vi "Teleop_Alternate.vi"(10 "Match Info":T1={"Autonomous Elapsed Seconds"=0.0, "TeleOp Elapsed Seconds"=0.0, "Disabled Elapsed Seconds"=0.0, "Visited Autonomous"=FALSE, "Visited TeleOp"=FALSE, "Visited Disabled"=FALSE, "Autonomous Settings"={"Autonomous Style"=enum."Independent", "VI Refnum"=refnum}}, 11 "Call Context":T2=enum."Stop") -> ()   [LabVIEW 2015]
doc: "This VI is called for each TeleOp packet received from the DS where the robot is not disabled. It is often used to read from the joysticks and update I/O or to update setpoints for timed control loops. It should complete and return within 20 milliseconds or it may miss DS packets."
uses:
  <vilib>/Rock Robotics/WPI/DriverStation/WPI_DriverStationDerivedRobotMode.ctl
  <vilib>/Rock Robotics/WPI/DriverStation/WPI_DriverStationMatch Info.ctl
  <vilib>/Rock Robotics/WPI/Solenoid/WPI_SolenoidValue.ctl
  Typedef/XBox Buttons.ctl
  Typedef/XBox Axis.ctl
  <vilib>/Rock Robotics/WPI/Utilities/WPI_GetSetVariantRefNum.vi
  <vilib>/Rock Robotics/Network Tables/NT Write Boolean Array.vi
  <vilib>/Rock Robotics/Network Tables/NT Write Numeric Array.vi
  Robot Global Data.vi
  <vilib>/Rock Robotics/WPI/RobotDrive/WPI_RobotDriveArcadeDrive_Standard(NoSaturation).vi
  <vilib>/Rock Robotics/Network Tables/NT Write Number.vi
  <vilib>/Rock Robotics/Network Tables/NT Write String.vi
  <vilib>/Rock Robotics/WPI/Solenoid/WPI_SolenoidSetEnum.vi
  ArmController/ArmController.lvlib
panel:
  in  "Reset":bool
  out "Shifts":i32
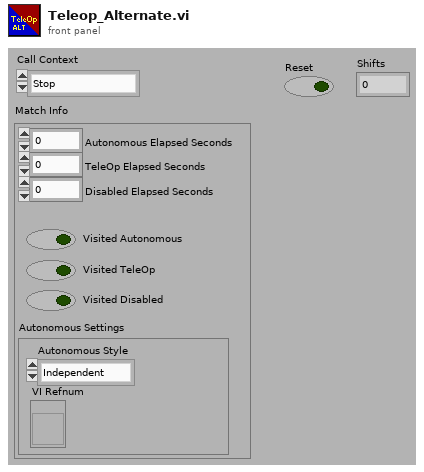
[diagram p1: front panel]
types:
  T1 = typedef "WPI_DriverStationMatch Info.ctl" = cluster{"Autonomous Elapsed Seconds":dbl, "TeleOp Elapsed Seconds":dbl, "Disabled Elapsed Seconds":dbl, "Visited Autonomous":bool, "Visited TeleOp":bool, "Visited Disabled":bool, "Autonomous Settings":cluster{"Autonomous Style":enum16{"Iterative", "Independent"}, "VI Refnum":refnum<vi>}}
  T2 = typedef "WPI_DriverStationDerivedRobotMode.ctl" = enum16{"Init", "Execute", "Stop"}
  T3 = typedef "WPI_SolenoidValue.ctl" = enum16{"Off", "On", "Forward", "Reverse"}
  T4 = typedef "WPI_JoystickDevRef.ctl" = cluster{"Device":T5}
  T5 = typedef "WPI_JoystickDeviceEnum.ctl" = enum16{"USB 0", "USB 1", "USB 2", "USB 3", "USB 4", "USB 5"}
  T6 = typedef "WPI_RobotDriveDevRef.ctl" = cluster{"DevStatus":errorcluster, "Motors[]":T7[], "Square Inputs":bool, "Max Output":dbl}
  T7 = typedef "WPI_MotorControlDeviceRef.ctl" = cluster{"DeviceStatus":errorcluster, "Type":T8, "PWM":cluster{"PWM Channel":T9, "DeadBand":T10}, "CAN":cluster{"Device Number":u8, "Control Mode":T11, "Semaphore":T12, "Max Vout":dbl, "TalonSRX Control Mode":T13}, "Invert":bool}
  T8 = typedef "WPI_MotorControlType.ctl" = enum16{"PWM", "CAN", "CANTalonSRX"}
  T9 = typedef "FPGA_DIOPWMChannel.ctl" = enum8{"PWM 0", "PWM 1", "PWM 2", "PWM 3", "PWM 4", "PWM 5", "PWM 6", "PWM 7", "PWM 8", "PWM 9", "PWM MXP 0", "PWM MXP 1", "PWM MXP 2", "PWM MXP 3", "PWM MXP 4", "PWM MXP 5", "PWM MXP 6", "PWM MXP 7", "PWM MXP 8", "PWM MXP 9", "Invalid"}
  T10 = typedef "WPI_PWMDeadband.ctl" = cluster{"Name":string, "maxPositivePwm":i32, "minPositivePwm":i32, "centerPwm":i32, "maxNegativePwm":i32, "minNegativePwm":i32, "angularRange":u16}
  T11 = typedef "WPI_CANJaguar_ControlMode.ctl" = enum8{"Percent VBus", "Current", "Speed", "Position", "Voltage"}
  T12 = typedef "Semaphore RefNum" = refnum<k1>
  T13 = typedef "WPI_CANTalonSRX_APIControlMode.ctl" = enum8{"Percent VBus", "Speed", "Position", "Slave", "Unchanged / Invalid", "Voltage Compensation", "Current", "Motion Profile"}
  T14 = typedef "XBox Axis.ctl" = enum16{"Left X", "Left Y", "Left Trigger", "Right Trigger", "Right X", "Right Y"}
  T15 = typedef "XBox Buttons.ctl" = enum16{"A", "B", "X", "Y", "Left Bumper", "Right Bumper", "Back", "Start", "Left Joystick", "Right Joystick"}
  T16 = typedef "ArmController.lvlib/ArmRef.ctl" = cluster{"Pot":T17, "ArmMotor":T7, "Queue":refnum<queue>, "Setpoint":dbl, "Manual":bool, "output range":cluster{"output high":dbl, "output low":dbl}, "PID gains":cluster{"proportional gain (Kc)":dbl, "integral time (Ti, min)":dbl, "derivative time (Td, min)":dbl}}
  T17 = typedef "WPI_PotentiometerDevRef.ctl" = cluster{"DevStatus":errorcluster, "Analog Channel":T18, "Invert Output":bool}
  T18 = typedef "FPGA_AIChannel.ctl" = enum8{"AI 0", "AI 1", "AI 2", "AI 3", "AI MXP 0", "AI MXP 1", "AI MXP 2", "AI MXP 3", "Invalid"}
  T19 = cluster{"Down":dbl, "Pickup":dbl, "Shoot":dbl, "Turtle":dbl, "Intake Transfer":dbl}
  T20 = typedef "WPI_SolenoidDevRef.ctl" = cluster{"DevStatus":errorcluster, "Pneumatics Control Module":u8, "Forward Solenoid Channel":T21, "Reverse Solenoid Channel":T21}
  T21 = typedef "WPI_SolenoidChannel.ctl" = enum8{"Solenoid 0", "Solenoid 1", "Solenoid 2", "Solenoid 3", "Solenoid 4", "Solenoid 5", "Solenoid 6", "Solenoid 7", "Invalid"}
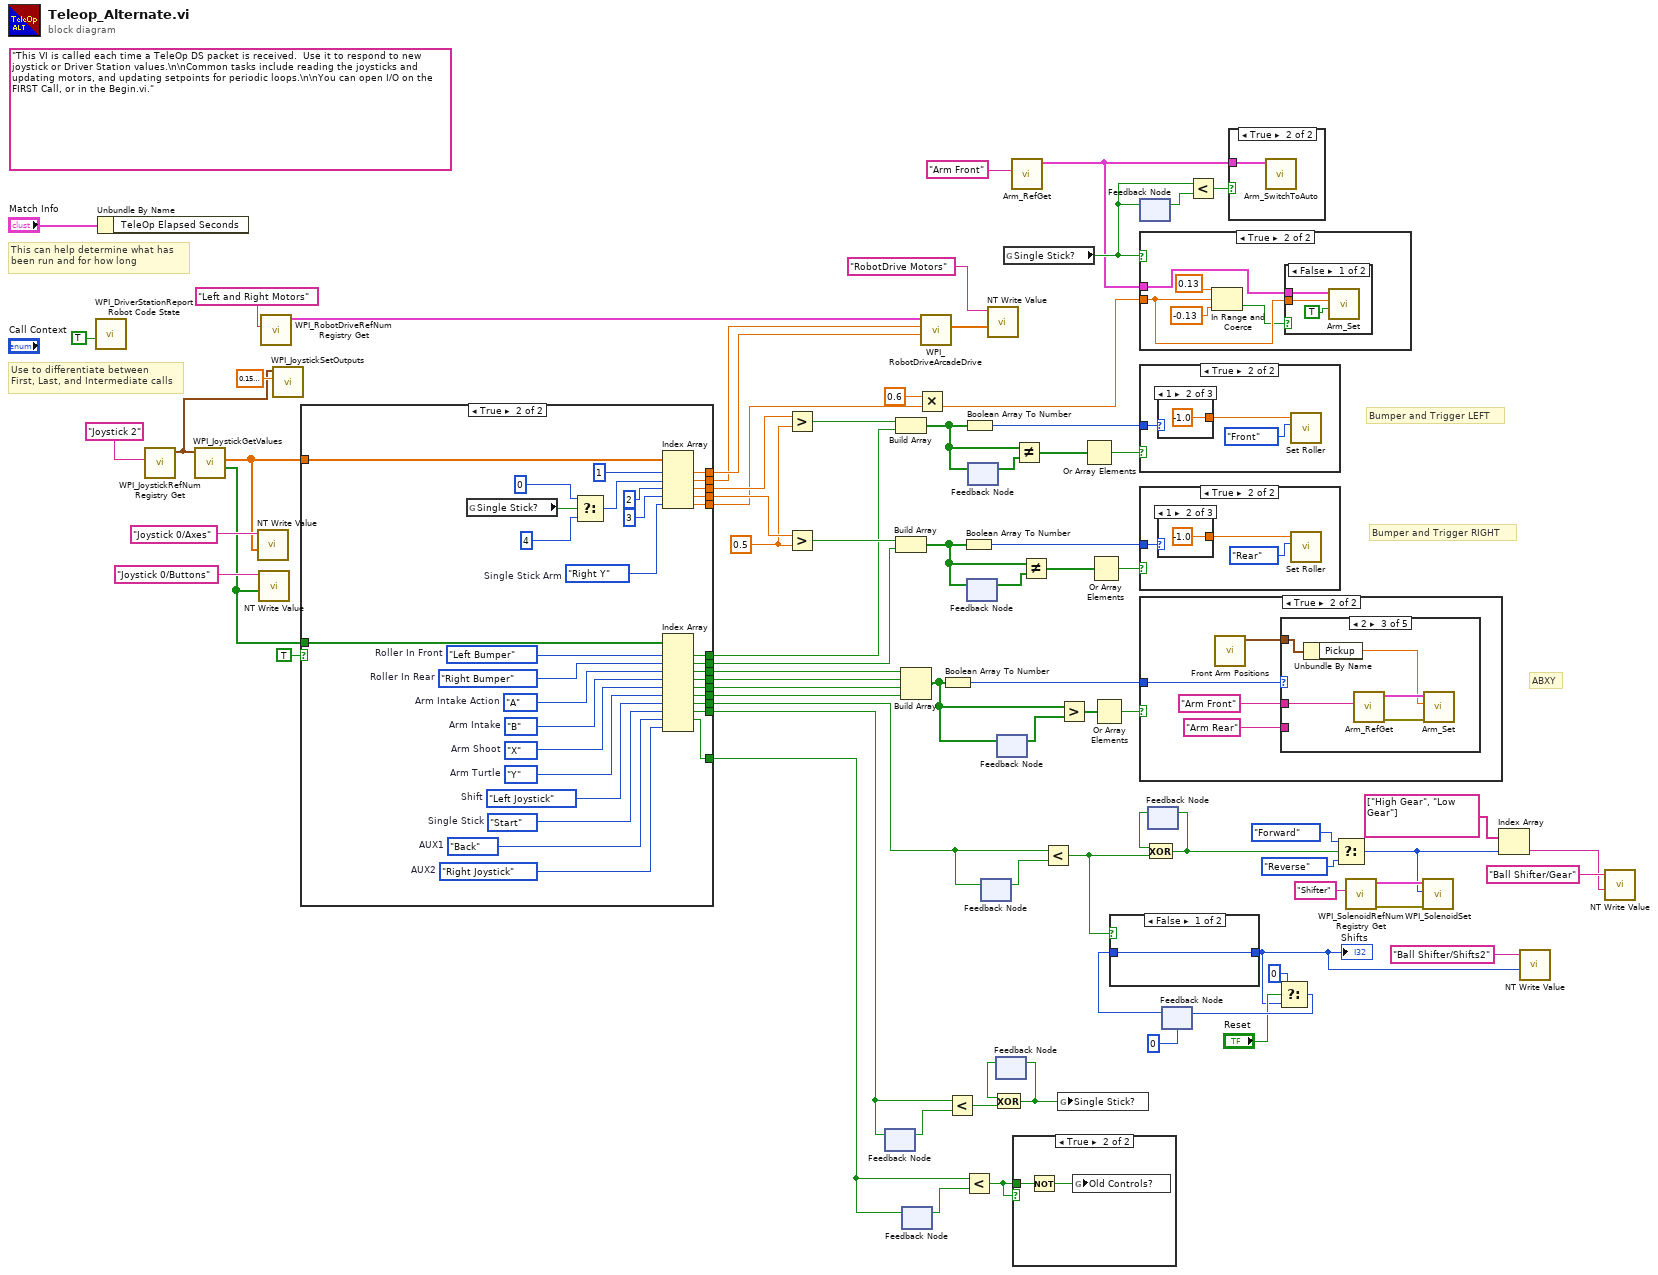
[diagram p0: block diagram]
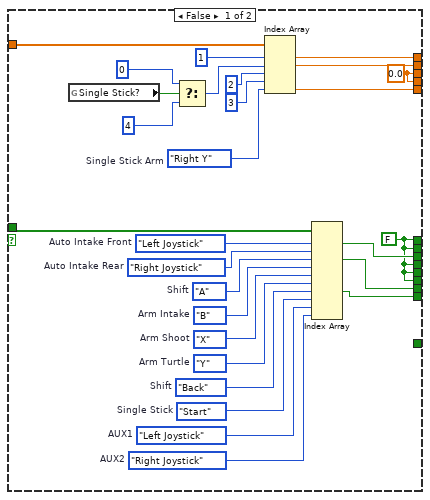
[diagram p3: hidden frame]
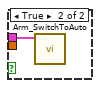
[diagram p6: hidden frame]
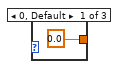
[diagram p8: hidden frame]
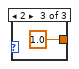
[diagram p9: hidden frame]
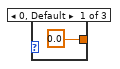
[diagram p11: hidden frame]
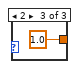
[diagram p12: hidden frame]
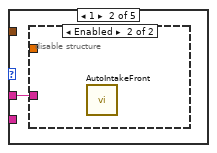
[diagram p15: hidden frame]
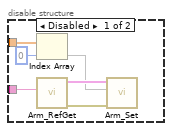
[diagram p16: hidden frame]
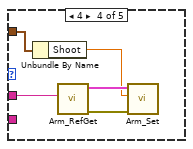
[diagram p17: hidden frame]
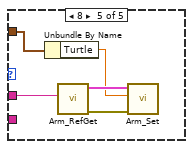
[diagram p18: hidden frame]
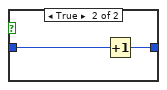
[diagram p19: hidden frame]
diagram:
  w44 = 0.5 ("x")
  (unwired) "This VI is called each time a TeleOp DS packet is received.  Use it to respond to new joystick or Driver Station values.\n\nCommon tasks include reading the joysticks and updating motors, and updating setpoints for periodic loops.\n\nYou can open I/O on the FIRST Call, or in the Begin.vi."
  # "ABXY"
  # "Bumper and Trigger RIGHT"
  # "Bumper and Trigger LEFT"
  # "Use to differentiate between\nFirst, Last, and Intermediate calls"
  # "This can help determine what has\nbeen run and for how long"
  n1 = call <vilib>:"WPI_DriverStationReport Robot Code State.vi"("TeleOp"=TRUE ("Autonomous")) -> ()  [unwired: 10 in, 1 out]
  n2 = Unbundle By Name("Match Info") -> ()  [unwired: 1 out]
  n3 = call <vilib>:"WPI_JoystickRefNum Registry Get.vi"("refnum name"="Joystick 2") -> ("JoystickDevRef"=w1:T4)  [unwired: 1 in, 9 out]
  n4 = call <vilib>:"WPI_JoystickGetValues.vi"("JoystickDevRef"=w1) -> ("Buttons"=w43:bool[], "Axes"=w47:dbl[])  [unwired: 6 in, 3 out]
  n5 = call-poly <vilib>:"NT Write Value.vi"("Numeric Array"=w47, "Name"="Joystick 0/Axes") -> ()  [unwired: 9 in, 1 out]
  n6 = call-poly <vilib>:"NT Write Value.vi"("Boolean Array"=w43, "Name"="Joystick 0/Buttons") -> ()  [unwired: 9 in, 1 out]
  n7 = call <vilib>:"WPI_RobotDriveRefNum Registry Get.vi"("refnum name"="Left and Right Motors") -> ("RobotDriveDevRef"=w78:T6)  [unwired: 1 in, 9 out]
  n8 = call <vilib>:"WPI_JoystickSetOutputs.vi"("Left Rumble"=sgl 0.15 ("Right Rumble"), "JoystickDevRef"=w1) -> ()  [unwired: 8 in, 2 out]
  n9 = case shown="True" TRUE {
    tunnel: [w86 w141] -> w76
    tunnel: [w85 w140] -> w73
    tunnel: [w81 w139] -> w67
    tunnel: w47 -> [w87 w138]
    tunnel: [w83 w134] -> w46
    tunnel: [w83 w133] -> w45
    tunnel: w43 -> [w97 w132]
    tunnel: [w82 w131] -> w40
    tunnel: [w82 w130] -> w39
    tunnel: [w96 w129] -> w38
    tunnel: [w82 w128] -> w37
    tunnel: [w82 w127] -> w36
    tunnel: [w82 w126] -> w35
    tunnel: [w80 w125] -> w20
    tunnel: [w84 w120] -> w13
    tunnel: [_ w108] -> w7
    frame False {
      w83 = 0.0 ("upper limit")
      w88 = XBox_Axis."Right Y"  # Single Stick Arm
      w107 = XBox_Buttons."Left Joystick"  # Auto Intake Front
      w106 = XBox_Buttons."Right Joystick"  # Auto Intake Rear
      w105 = XBox_Buttons."A"  # Shift
      w104 = XBox_Buttons."B"  # Arm Intake
      w103 = XBox_Buttons."X"  # Arm Shoot
      w102 = XBox_Buttons."Y"  # Arm Turtle
      w100 = XBox_Buttons."Back"  # Shift
      w99 = XBox_Buttons."Start"  # Single Stick
      w101 = XBox_Buttons."Right Joystick"  # AUX2
      w98 = XBox_Buttons."Left Joystick"  # AUX1
      w82 = FALSE
      n10 = global read "Robot Global Data.vi" "Single Stick?"() -> (w92:bool)
      n11 = Select(t=0 ("index"), s=w92, f=4 ("index")) -> (s? t:f=w89:i32)
      n12 = Index Array(array=w87, index #1=1 ("index"), index #2=w89, index #3=2 ("index"), index #4=3 ("index"), index #5=w88) -> (element #1=w86:dbl, element #2=w85:dbl, element #5=w84:dbl)  [unwired: 2 out]
      n13 = Index Array(array=w97, index #1=w107, index #2=w106, index #3=w105, index #4=w104, index #5=w103, index #6=w102, index #7=w100, index #8=w99, index #9=w98, index #10=w101) -> (element #1=w96:bool, element #3=w81:bool, element #7=w80:bool)  [unwired: 7 out]
    }
    frame True {
      w109 = XBox_Axis."Right Y"  # Single Stick Arm
      w110 = XBox_Buttons."Left Bumper"  # Roller In Front
      w111 = XBox_Buttons."Right Bumper"  # Roller In Rear
      w112 = XBox_Buttons."A"  # Arm Intake Action
      w113 = XBox_Buttons."B"  # Arm Intake
      w114 = XBox_Buttons."X"  # Arm Shoot
      w115 = XBox_Buttons."Y"  # Arm Turtle
      w117 = XBox_Buttons."Left Joystick"  # Shift
      w118 = XBox_Buttons."Start"  # Single Stick
      w116 = XBox_Buttons."Right Joystick"  # AUX2
      w119 = XBox_Buttons."Back"  # AUX1
      n14 = global read "Robot Global Data.vi" "Single Stick?"() -> (w124:bool)
      n15 = Select(t=0 ("index"), s=w124, f=4 ("index")) -> (s? t:f=w121:i32)
      n16 = Index Array(array=w138, index #1=1 ("index"), index #2=w121, index #3=2 ("index"), index #4=3 ("index"), index #5=w109) -> (element #1=w141:dbl, element #2=w140:dbl, element #3=w134:dbl, element #4=w133:dbl, element #5=w120:dbl)
      n17 = Index Array(array=w132, index #1=w110, index #2=w111, index #3=w112, index #4=w113, index #5=w114, index #6=w115, index #7=w117, index #8=w118, index #9=w119, index #10=w116) -> (element #1=w131:bool, element #2=w130:bool, element #3=w129:bool, element #4=w128:bool, element #5=w127:bool, element #6=w126:bool, element #7=w139:bool, element #8=w125:bool, element #9=w108:bool)  [unwired: 1 out]
    }
  }
  n18 = Greater?(x=w46, y=w44) -> (0:w41:bool)
  n19 = Greater?(x=w45, y=w44) -> (0:w42:bool)
  n20 = feedback #1() -> (w21:bool)  [unwired: 1 in]
  n21 = feedback-in #1(w20) -> ()
  n22 = Build Array(w41, w40) -> (w32:bool[])
  n23 = Build Array(w42, w39) -> (w26:bool[])
  n24 = Build Array(w38, w37, w36, w35) -> (w55:bool[])
  n25 = feedback #2() -> (w6:bool)  [unwired: 1 in]
  n26 = feedback-in #2(w7) -> ()
  n27 = Multiply(x=0.6, y=w13) -> (x*y=w4:dbl)
  n28 = call-poly <vilib>:"WPI_RobotDriveArcadeDrive.vi"("Y axis value"=w76, "X axis value"=w73, "RobotDriveDevRef"=w78) -> ("Motor Values"=w75:dbl[])  [unwired: 6 in, 2 out]
  n29 = Boolean Array To Number(Boolean array=w55) -> (number=w52:u32)
  n30 = Less?(x=w20, y=w21) -> (x < y?=w23:bool)
  n31 = Boolean Array To Number(Boolean array=w26) -> (number=w24:u32)
  n32 = Less?(x=w7, y=w6) -> (x < y?=w5:bool)
  n33 = Boolean Array To Number(Boolean array=w32) -> (number=w57:u32)
  n34 = feedback #3() -> (w28:bool[])  [unwired: 1 in]
  n35 = feedback-in #3(w26) -> ()
  n36 = feedback-in #4(w32) -> ()
  n37 = feedback #4() -> (w31:bool[])  [unwired: 1 in]
  n38 = feedback #5() -> (w69:bool)  [unwired: 1 in]
  n39 = feedback-in #5(w67) -> ()
  n40 = call-poly <vilib>:"NT Write Value.vi"("Numeric Array"=w75, "Name"="RobotDrive Motors") -> ()  [unwired: 9 in, 1 out]
  n41 = feedback #6() -> (w22:bool)  [unwired: 1 in]
  n42 = Exclusive Or(1:w23, 2:w22) -> (0:w19:bool)
  n43 = feedback-in #6(w19) -> ()
  n44 = feedback #7() -> (w56:bool[])  [unwired: 1 in]
  n45 = feedback-in #7(w55) -> ()
  n46 = global read "Robot Global Data.vi" "Single Stick?"() -> (w17:bool)
  n47 = call "Arm_RefGet.vi"("refnum name"="Arm Front") -> ("ArmRef"=w14:T16)  [unwired: 9 in, 1 out]
  n48 = case shown="True" w5 {
    tunnel: w5 -> [_ w143]
    frame False {
    }
    frame True {
      n49 = Not(x=w143) -> (.not. x?=w142:bool)
      n50 = global write "Robot Global Data.vi" "Old Controls?"(w142) -> ()
    }
  }
  n51 = Not Equal?(x=w32, y=w31) -> (x != y?=w30:bool[])
  n52 = Not Equal?(x=w26, y=w28) -> (x != y?=w27:bool[])
  n53 = Less?(x=w67, y=w69) -> (x < y?=w61:bool)
  n54 = global write "Robot Global Data.vi" "Single Stick?"(w19) -> ()
  n55 = Greater?(x=w55, y=w56) -> (0:w54:bool[])
  n56 = Or Array Elements(Boolean array=w30) -> (logical OR=w29:bool)
  n57 = Or Array Elements(Boolean array=w27) -> (logical OR=w25:bool)
  n58 = Or Array Elements(Boolean array=w54) -> (logical OR=w53:bool)
  n59 = feedback #8() -> (w18:bool)  [unwired: 1 in]
  n60 = feedback-in #8(w17) -> ()
  n61 = case shown="True" w17 {
    tunnel: w14 -> [_ w146]
    tunnel: w4 -> [_ w145]
    frame False {
    }
    frame True {
      n62 = In Range and Coerce(upper limit=0.13, x=w145, lower limit=-0.13) -> (In Range?=w144:bool)  [unwired: 1 out]
      n63 = case shown="False" w144 {
        tunnel: w146 -> [w151 w152]
        tunnel: w145 -> [w150 _]
        frame False {
          n64 = call "Arm_Set.vi"("Manual Control"=TRUE, "Value"=w150, "ArmRef in"=w151) -> ()  [unwired: 7 in, 2 out]
        }
        frame True {
          n65 = call "Arm_SwitchToAuto.vi"("ArmRef in"=w152) -> ()  [unwired: 9 in, 2 out]
        }
      }
    }
  }
  n66 = case shown="True" w29 {
    tunnel: w57 -> [_ w155]
    frame False {
    }
    frame True {
      n67 = case shown="1" w155 {
        tunnel: [0.0 ("Speed") -1.0 ("Speed") 1.0 ("Speed")] -> w154
        frame 0, Default {
        }
        frame 1 {
        }
        frame 2 {
        }
      }
      n68 = call "Set Roller.vi"("Intake"=enum16{"Front", "Rear"}."Front", "Speed"=w154) -> ()  [unwired: 10 in]
    }
  }
  n69 = case shown="True" w25 {
    tunnel: w24 -> [_ w161]
    frame False {
    }
    frame True {
      n70 = case shown="1" w161 {
        tunnel: [0.0 ("Speed") -1.0 ("Speed") 1.0 ("Speed")] -> w160
        frame 0, Default {
        }
        frame 1 {
        }
        frame 2 {
        }
      }
      n71 = call "Set Roller.vi"("Intake"=enum16{"Front", "Rear"}."Rear", "Speed"=w160) -> ()  [unwired: 10 in]
    }
  }
  n72 = case shown="True" w53 {
    tunnel: w52 -> [_ w168]
    frame False {
    }
    frame True {
      n73 = call "Front Arm Positions.vi"() -> ("Front Arm"=w165:T19)  [unwired: 10 in, 1 out]
      n74 = case shown="2" w168 {
        tunnel: "Arm Front" ("refnum name") -> [_ w169 w180 w183 w188]
        tunnel: "Arm Rear" ("refnum name") -> [_ _ _ _ _]
        tunnel: w165 -> [_ _ w177 w182 w187]
        frame 0, Default {
        }
        frame 1 {
          n75 = disable-structure shown="Enabled" {
            disable-tunnel: w169 -> [w175 _]
            disable-tunnel: _ -> [w171 _]
            frame Disabled {
              n76 = Index Array(array=w171, index=0) -> (element=w172)
              n77 = call "Arm_RefGet.vi"("refnum name"=w175) -> ("error out"=w174:errorcluster, "ArmRef"=w173:T16)  [unwired: 9 in]
              n78 = call "Arm_Set.vi"("error in (no error)"=w174, "Value"=w172, "ArmRef in"=w173) -> ()  [unwired: 7 in, 2 out]
            }
            frame Enabled {
              n79 = call "AutoIntakeFront.vi"() -> ()  [unwired: 12 in]
            }
          }
        }
        frame 2 {
          n80 = Unbundle By Name(w177) -> ("Pickup"=w176:dbl)
          n81 = call "Arm_RefGet.vi"("refnum name"=w180) -> ("error out"=w179:errorcluster, "ArmRef"=w178:T16)  [unwired: 9 in]
          n82 = call "Arm_Set.vi"("error in (no error)"=w179, "Value"=w176, "ArmRef in"=w178) -> ()  [unwired: 7 in, 2 out]
        }
        frame 4 {
          n83 = Unbundle By Name(w182) -> ("Shoot"=w181:dbl)
          n84 = call "Arm_RefGet.vi"("refnum name"=w183) -> ("error out"=w185:errorcluster, "ArmRef"=w184:T16)  [unwired: 9 in]
          n85 = call "Arm_Set.vi"("error in (no error)"=w185, "Value"=w181, "ArmRef in"=w184) -> ()  [unwired: 7 in, 2 out]
        }
        frame 8 {
          n86 = Unbundle By Name(w187) -> ("Turtle"=w186:dbl)
          n87 = call "Arm_RefGet.vi"("refnum name"=w188) -> ("error out"=w190:errorcluster, "ArmRef"=w189:T16)  [unwired: 9 in]
          n88 = call "Arm_Set.vi"("error in (no error)"=w190, "Value"=w186, "ArmRef in"=w189) -> ()  [unwired: 7 in, 2 out]
        }
      }
    }
  }
  n89 = feedback #9() -> (w68:bool)  [unwired: 1 in]
  n90 = Exclusive Or(1:w61, 2:w68) -> (0:w66:bool)
  n91 = feedback-in #9(w66) -> ()
  n92 = feedback #10(0) -> (w62:i32)
  n93 = case shown="False" w61 {
    tunnel: w62 -> [w191 w193]
    tunnel: [w191 w192] -> w34
    frame False {
    }
    frame True {
      n94 = Increment(x=w193) -> (x+1=w192:i32)
    }
  }
  "Shifts" <- w34
  n95 = Less?(x=w17, y=w18) -> (x < y?=w16:bool)
  n96 = case shown="True" w16 {
    tunnel: w14 -> [_ w194]
    frame False {
    }
    frame True {
      n97 = call "Arm_SwitchToAuto.vi"("ArmRef in"=w194) -> ()  [unwired: 9 in, 2 out]
    }
  }
  n98 = Select(t=0, s="Reset", f=w34) -> (s? t:f=w59:i32)
  n99 = feedback-in #10(w59) -> ()
  n100 = Select(t=WPI_SolenoidValue."Forward" ("Value"), s=w66, f=WPI_SolenoidValue."Reverse" ("Value")) -> (s? t:f=w10:T3)
  n101 = call <vilib>:"WPI_SolenoidRefNum Registry Get.vi"("refnum name"="Shifter") -> ("error out"=w70:errorcluster, "SolenoidDevRef"=w71:T20)  [unwired: 9 in]
  n102 = call-poly <vilib>:"WPI_SolenoidSet.vi"("error in (no error)"=w70, "Value"=w10, "SolenoidDevRef"=w71) -> ()  [unwired: 7 in, 2 out]
  n103 = Index Array(array=string[] ["High Gear", "Low Gear"], index=w10) -> (element=w9:string)
  n104 = call-poly <vilib>:"NT Write Value.vi"("Numeric"=w34, "Name"="Ball Shifter/Shifts2") -> ()  [unwired: 9 in, 1 out]
  n105 = call-poly <vilib>:"NT Write Value.vi"("String"=w9, "Name"="Ball Shifter/Gear") -> ()  [unwired: 9 in, 1 out]
